vi "AR-DO-test.vi"() -> ()   [LabVIEW 2021]
panel:
  out "Data 2":dbl[](array[numeric]) format="%0.2f"
  out "Data":bool[](array[boolean])
  in  "stop":bool
  out "error out":errorcluster
  in  "data":bool
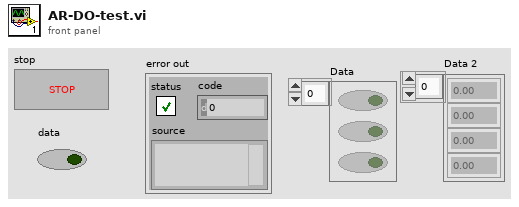
[diagram p1: front panel]
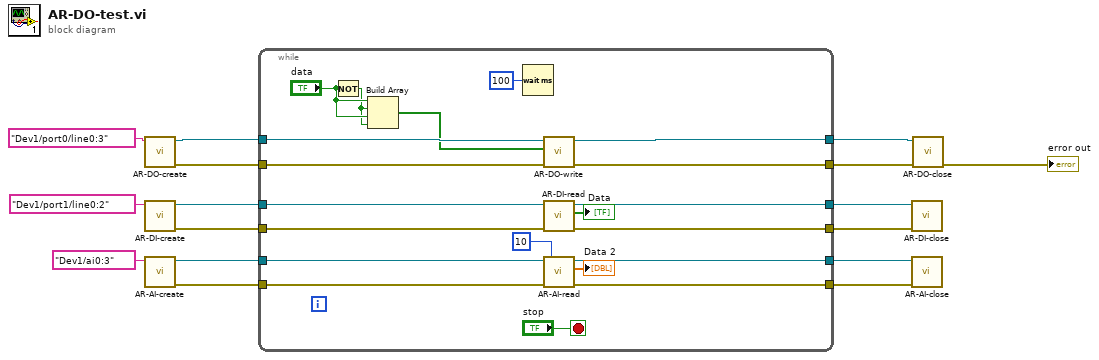
[diagram p0: block diagram]
diagram:
  n1 = call "AR-DO-create.vi"("lines"=tag "Dev1/port0/line0:3") -> ("error out"=w11:errorcluster, "DO task out"=w12:refnum<k21>)  [unwired: 9 in]
  n2 = call "AR-DI-create.vi"("lines"=tag "Dev1/port1/line0:2") -> ("error out"=w10:errorcluster, "DI task out"=w7:refnum<k21>)  [unwired: 9 in]
  n3 = call "AR-AI-create.vi"("lines"=tag "Dev1/ai0:3") -> ("error out"=w5:errorcluster, "AI task out"=w4:refnum<k21>)  [unwired: 9 in]
  n4 = while {
    tunnel: w12 -> [w34]
    tunnel: w11 -> [w33]
    tunnel: [w28] -> w14
    tunnel: [w29] -> w13
    tunnel: w10 -> [w27]
    tunnel: [w26] -> w9
    tunnel: w7 -> [w25]
    tunnel: [w24] -> w6
    tunnel: w5 -> [w22]
    tunnel: w4 -> [w21]
    tunnel: [w20] -> w3
    tunnel: [w19] -> w2
    stop <- "stop" stop-if-true
    n5 = Not(x="data") -> (.not. x?=w31:bool)
    n6 = Build Array("data", w31, "data", w31) -> (w30:bool[])
    n7 = Wait (ms)(milliseconds to wait=u32 100) -> ()  [unwired: 1 out]
    n8 = call "AR-DO-write.vi"("error in (no error)"=w33, "Data"=w30, "DO task in"=w34) -> ("error out"=w28:errorcluster, "DO task out"=w29:refnum<k21>)  [unwired: 7 in]
    n9 = call "AR-DI-read.vi"("error in"=w27, "DI task in"=w25) -> ("error out"=w26:errorcluster, "Data"=→"Data":bool[], "DI task out"=w24:refnum<k21>)  [unwired: 7 in]
    n10 = call "AR-AI-read.vi"("number of samples"=10, "error in"=w22, "AI task in"=w21) -> ("error out"=w20:errorcluster, "Data"=→"Data 2":dbl[], "AI task out"=w19:refnum<k21>)  [unwired: 6 in]
  }
  n11 = call "AR-DI-close.vi"("error in (no error)"=w9, "DI task in"=w6) -> ()  [unwired: 9 in, 1 out]
  n12 = call "AR-AI-close.vi"("error in (no error)"=w3, "AI task in"=w2) -> ()  [unwired: 9 in, 1 out]
  n13 = call "AR-DO-close.vi"("error in (no error)"=w14, "DO task in"=w13) -> ("error out"=→"error out":errorcluster)  [unwired: 9 in]
